vi "ReplaceControlNode.vi"(5 "Old File Name":string, 7 "New File Name":string, 8 "error in (no error)":errorcluster, 11 "VI Refnum In":refnum<vi>) -> (0 "error out":errorcluster, 3 "VI Refnum Out":refnum<vi>, 4 "Replaced":bool)   [LabVIEW 2024]
uses:
  <vilib>/Utility/traverseref.llb/TRef TravTarget.ctl
  <vilib>/Utility/traverseref.llb/VI Scripting - Traverse.lvlib
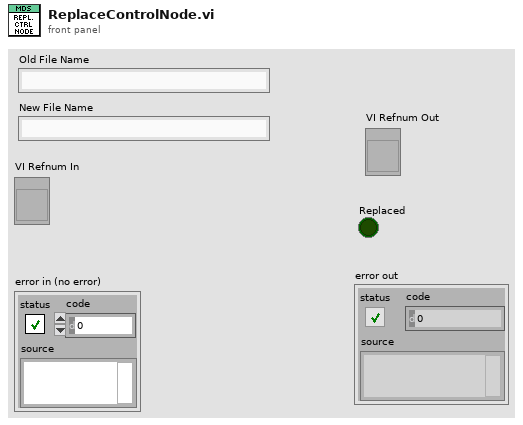
[diagram p1: front panel]
types:
  T1 = typedef "TRef TravTarget.ctl" = enum16{"FP", "BD", "Other"}
  T2 = enum32{"not a typedef", "typedef", "strict typedef", "class private data"}
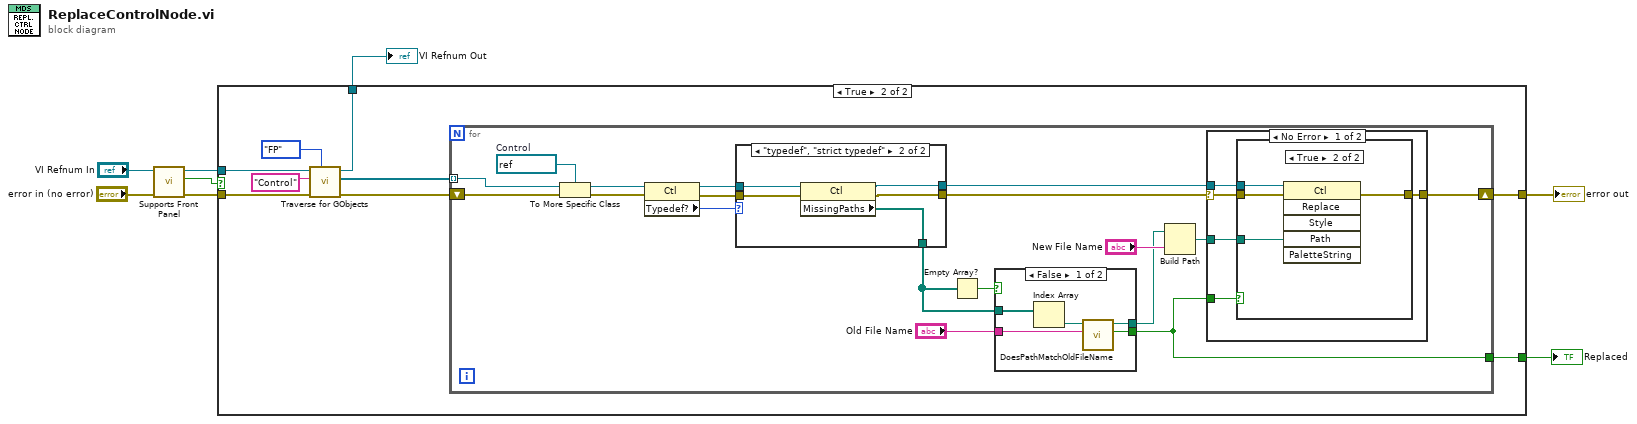
[diagram p0: block diagram]
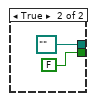
[diagram p3: hidden frame]
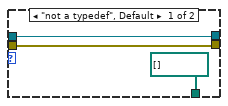
[diagram p4: hidden frame]
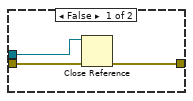
[diagram p5: hidden frame]
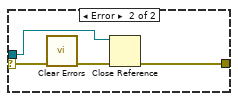
[diagram p6: hidden frame]
diagram:
  n1 = call "Supports Front Panel.vi"("error in (no error)"="error in (no error)", "vi in"="VI Refnum In") -> ("error out"=w2:errorcluster, "has front panel"=w1:bool, "vi out"=w3:refnum<vi>)  [unwired: 7 in]
  n2 = case shown="True" w1 {
    tunnel: [w9 w16] -> w8
    tunnel: [_ w15] -> w7
    tunnel: w2 -> [w10 w14]
    tunnel: w3 -> [w9 w13]
    tunnel: [w10 w11] -> w6
    frame False {
    }
    frame True {
      n3 = call <vilib>:"Traverse for GObjects.vi"("Traverse Target"=TRef_TravTarget."FP", "error in (no error)"=w14, "Class Name"="Control", "VI Refnum"=w13) -> ("error out"=w19:errorcluster, "References"=w12:refnum<vi>[], "dup VI Refnum"=w16:refnum<vi>)  [unwired: 4 in, 1 out]
      n4 = for {
        shift-right: [w35] -> w11
        shift-left: w19 -> [w36]
        tunnel: w12 -> [w37] mode=indexing
        tunnel: [w23] -> w15
        w32 = refnum<vi> refnum  # Control
        n5 = To More Specific Class(target class=w32, reference=w37, error in=w36) -> (specific class reference=w31:refnum<vi>, error out=w30:errorcluster)
        n6 = property class="Ctl"(reference=w31, error in=w30) -> (reference out=w27:refnum<vi>, error out=w29:errorcluster, "Typedef?"=w25:T2)
        n7 = case shown="\"typedef\", \"strict typedef\"" w25 {
          tunnel: [path[] [] ("MissingPaths") w52] -> w20
          tunnel: w29 -> [w45 w51]
          tunnel: [w45 w50] -> w28
          tunnel: w27 -> [w46 w49]
          tunnel: [w46 w48] -> w26
          frame "not a typedef", Default {
          }
          frame "typedef", "strict typedef" {
            n8 = property class="Ctl"(reference=w49, error in=w51) -> (reference out=w48:refnum<vi>, error out=w50:errorcluster, "MissingPaths"=w52:path[])
          }
        }
        n9 = Empty Array?(array=w20) -> (empty?=w21:bool)
        n10 = case shown="False" w21 {
          tunnel: w20 -> [w42 _]
          tunnel: "Old File Name" -> [w41 _]
          tunnel: [w39 FALSE ("Match Found")] -> w23
          tunnel: [w38 path "" ("Parent Directory")] -> w22
          frame False {
            n11 = Index Array(array=w42) -> (element=w40:path)  [unwired: 1 in]
            n12 = call "DoesPathMatchOldFileName.vi"("Old File Name"=w41, "File Path"=w40) -> ("Match Found"=w39:bool, "Parent Directory"=w38:path)  [unwired: 8 in]
          }
          frame True {
          }
        }
        n13 = Build Path(base path=w22, name or relative path="New File Name") -> (appended path=w34:path)
        n14 = case shown="No Error" w28 {
          selector: w28 -> [w53 w68]
          tunnel: w34 -> [w57 _]
          tunnel: w23 -> [w56 _]
          tunnel: [w55 w66] -> w35
          tunnel: w26 -> [w54 w65]
          frame No Error {
            n15 = case shown="True" w56 {
              tunnel: w57 -> [_ w64]
              tunnel: w53 -> [w60 w63]
              tunnel: [w59 w61] -> w55
              tunnel: w54 -> [w58 w62]
              frame False {
                n16 = Close Reference(reference=w58, error in (no error)=w60) -> (error out=w59:errorcluster)
              }
              frame True {
                n17 = invoke class="Ctl" method="Replace"(reference=w62, error in=w63, "Path"=w64) -> (error out=w61:errorcluster)  [unwired: 3 in, 5 out]
              }
            }
          }
          frame Error {
            n18 = call <vilib>:"Clear Errors.vi"("error in (no error)"=w68) -> ("error out"=w67:errorcluster)  [unwired: 5 in, 1 out]
            n19 = Close Reference(reference=w65, error in (no error)=w67) -> (error out=w66:errorcluster)
          }
        }
      }
    }
  }
  "error out" <- w6
  "VI Refnum Out" <- w8
  "Replaced" <- w7
